vi "LoadSerialNumbers.vi"(8 "error in":errorcluster, 11 "License":string="2") -> (0 "error out":errorcluster, 2 "Serials":string[](array[string]), 3 "ID":string)   [LabVIEW 2013, in "main.lvlib"]
uses:
  main.lvlib
panel:
  out "JSON string":string
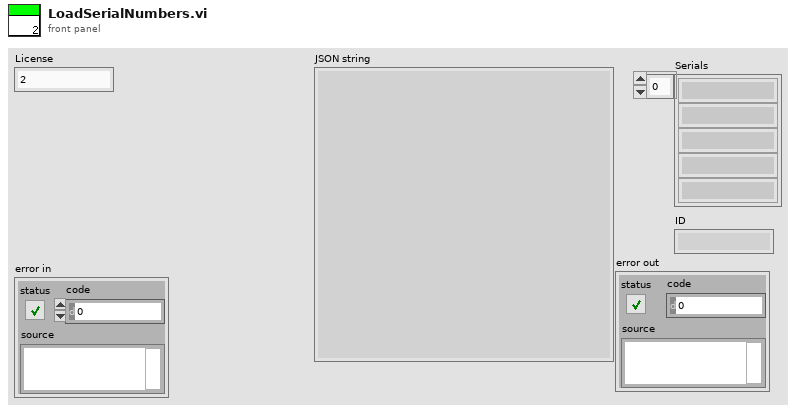
[diagram p1: front panel]
types:
  T1 = cluster{"LicenseID":string, "Serials":string[], "ID":string}[]
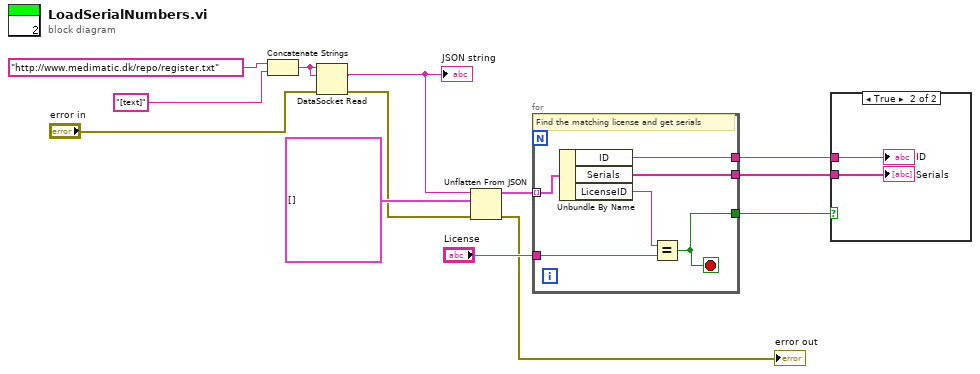
[diagram p0: block diagram]
diagram:
  n1 = Concatenate Strings("http://www.medimatic.dk/repo/register.txt" ("connection in"), "[text]") -> (w1:string)
  n2 = DataSocket Read(8:"error in", 10:w1, 11:w1) -> (0:w4:errorcluster, 2:w5:string)  [unwired: 2 in, 5 out]
  "JSON string" <- w5
  n3 = Unflatten From JSON(JSON string=w5, type and defaults=T1 [], error in (no error)=w4) -> (value=w12:T1, error out=→"error out":errorcluster)  [unwired: 4 in]
  n4 = for {
    tunnel: w12 -> [w19] mode=indexing
    tunnel: [w17] -> w11
    tunnel: "License" -> [w16]
    tunnel: [w15] -> w9
    tunnel: [w14] -> w7
    stop <- w14 stop-if-true
    # "Find the matching license and get serials"
    n5 = Unbundle By Name(w19) -> ("ID"=w15:string, "Serials"=w17:string[], "LicenseID"=w18:string)
    n6 = Equal?(x=w18, y=w16) -> (x = y?=w14:bool)
  }
  n7 = case shown="True" w7 {
    tunnel: w11 -> [_ w21]
    tunnel: w9 -> [_ w20]
    frame False {
    }
    frame True {
      "Serials" <- w21
      "ID" <- w20
    }
  }
